vi "2D array sort with key.vi"(1 "ascending":bool, 2 "key row":dbl, 3 "input":dbl[][](array[numeric])) -> (0 "output":dbl[][](array[numeric]))   [LabVIEW 2019]
panel:
  out "size(s)":i32[](array[numeric])
  # "descending"
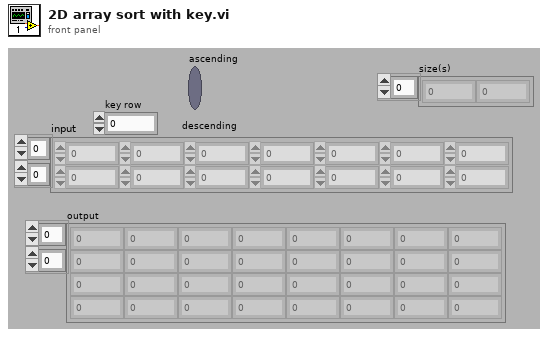
[diagram p1: front panel]
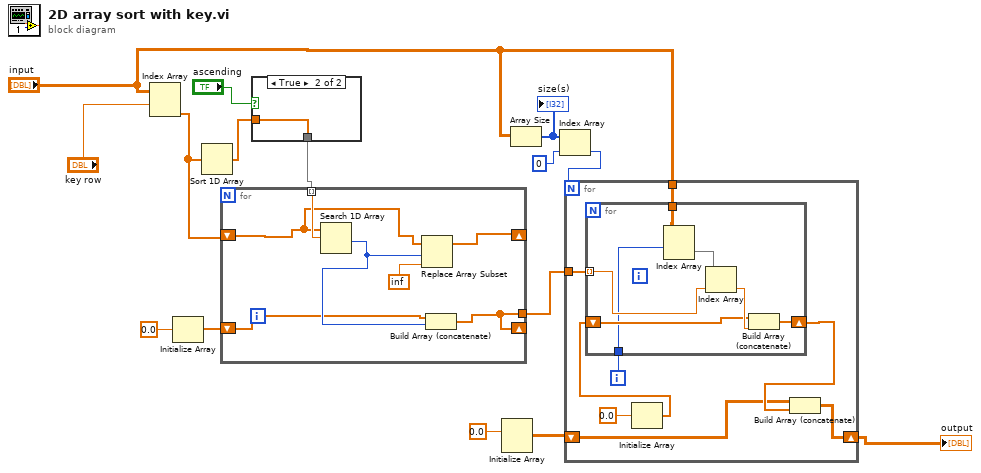
[diagram p0: block diagram]
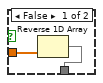
[diagram p2: hidden frame]
diagram:
  n1 = Index Array(array="input", index (row)="key row") -> (element=w12:dbl[])  [unwired: 1 in]
  n2 = Initialize Array(0.0 ("element")) -> (w13:dbl[])  [unwired: 1 out]
  n3 = Sort 1D Array(array=w12) -> (sorted array=w5:dbl[])
  n4 = case shown="True" "ascending" {
    tunnel: [w16 w18] -> w6
    tunnel: w5 -> [w17 w18]
    frame False {
      n5 = Reverse 1D Array(array=w17) -> (reversed array=w16:dbl[])
    }
    frame True {
    }
  }
  n6 = for {
    tunnel: w6 -> [w25] mode=indexing
    tunnel: [w21] -> w15
    shift-right: [w22] -> _
    shift-left: w12 -> [w23]
    shift-right: [w21] -> _
    shift-left: w13 -> [w20]
    n7 = Search 1D Array(1D array=w23, element=w25) -> (index of element=w24:i32)  [unwired: 1 out]
    n8 = Replace Array Subset(array=w23, new element=inf, index=w24) -> (w22:dbl[])
    n9 = Build Array (concatenate)(w20, w24) -> (w21:dbl[])
  }
  n10 = Initialize Array(0.0 ("element")) -> (w7:dbl[][])  [unwired: 2 out]
  n11 = Array Size(array="input") -> (size(s)=w11:i32[])
  "size(s)" <- w11
  n12 = Index Array(array=w11, index=0) -> (element=w9:i32)
  n13 = for {
    N: w9 -> [_]
    tunnel: w15 -> [w33]
    tunnel: "input" -> [w32]
    shift-right: [w26] -> w1
    shift-left: w7 -> [w27]
    i -> [w31]
    n14 = Initialize Array(0.0 ("element")) -> (w29:dbl[])  [unwired: 1 out]
    n15 = for {
      shift-right: [w35] -> w28
      shift-left: w29 -> [w36]
      tunnel: w33 -> [w38] mode=indexing
      tunnel: w32 -> [w40]
      tunnel: w31 -> [w34]
      n16 = Index Array(array=w40, index (row)=w34) -> (element=w39:dbl[])  [unwired: 1 in]
      n17 = Index Array(array=w39, index=w38) -> (element=w37:dbl)
      n18 = Build Array (concatenate)(w36, w37) -> (w35:dbl[])
    }
    n19 = Build Array (concatenate)(w27, w28) -> (w26:dbl[][])
  }
  "output" <- w1
